vi "SFC_Rep Maintenance.vi"(5 "tblName":string, 6 "OperatorName":string, 7 "ModuleName":string, 8 "error in (no error)":errorcluster caption="错误输入（无错误）", 9 "Type":string, 10 ".NET:System.Data.DataSet":T1={"CaseSensitive"=FALSE, "Container"=refnum, "DataSetName"="", "DefaultViewManager"=refnum, "DesignMode"=FALSE, "EnforceConstraints"=FALSE, "ExtendedProperties"=refnum, "HasErrors"=FALSE, "IsInitialized"=FALSE, "Locale"=refnum, "Namespace"="", "Prefix"="", "Relations"=refnum, "RemotingFormat"=0, "SchemaSerializationMode"=1, "Site"=refnum, "Tables"=refnum} {"SchemaSerializationMode" items=["IncludeSchema"=1, "ExcludeSchema"=2]; "RemotingFormat" items=["Xml", "Binary"]}, 11 "Traceability 引用句柄":refnum<k24>) -> (0 "error out":errorcluster caption="错误输出", 2 ".NET:System.Data.DataSet":T1={"CaseSensitive"=FALSE, "Container"=refnum, "DataSetName"="", "DefaultViewManager"=refnum, "DesignMode"=FALSE, "EnforceConstraints"=FALSE, "ExtendedProperties"=refnum, "HasErrors"=FALSE, "IsInitialized"=FALSE, "Locale"=refnum, "Namespace"="", "Prefix"="", "Relations"=refnum, "RemotingFormat"=0, "SchemaSerializationMode"=1, "Site"=refnum, "Tables"=refnum} {"SchemaSerializationMode" items=["IncludeSchema"=1, "ExcludeSchema"=2]; "RemotingFormat" items=["Xml", "Binary"]}, 3 "Traceability 引用句柄输出":refnum<k24>)   [LabVIEW 2014, in "Traceability.lvlib"]
uses:
  Traceability.lvlib
  Traceability.dll
  System.Data
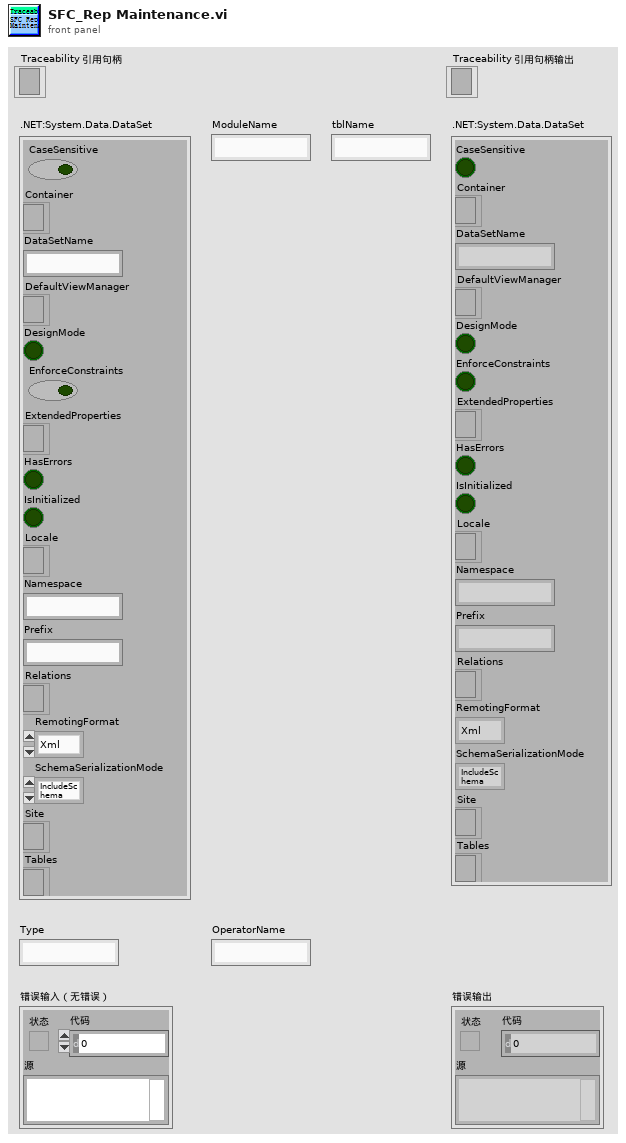
[diagram p1: front panel]
types:
  T1 = cluster{"CaseSensitive":bool, "Container":refnum<k24>, "DataSetName":string, "DefaultViewManager":refnum<k24>, "DesignMode":bool, "EnforceConstraints":bool, "ExtendedProperties":refnum<k24>, "HasErrors":bool, "IsInitialized":bool, "Locale":refnum<k24>, "Namespace":string, "Prefix":string, "Relations":refnum<k24>, "RemotingFormat":i32, "SchemaSerializationMode":i32, "Site":refnum<k24>, "Tables":refnum<k24>}
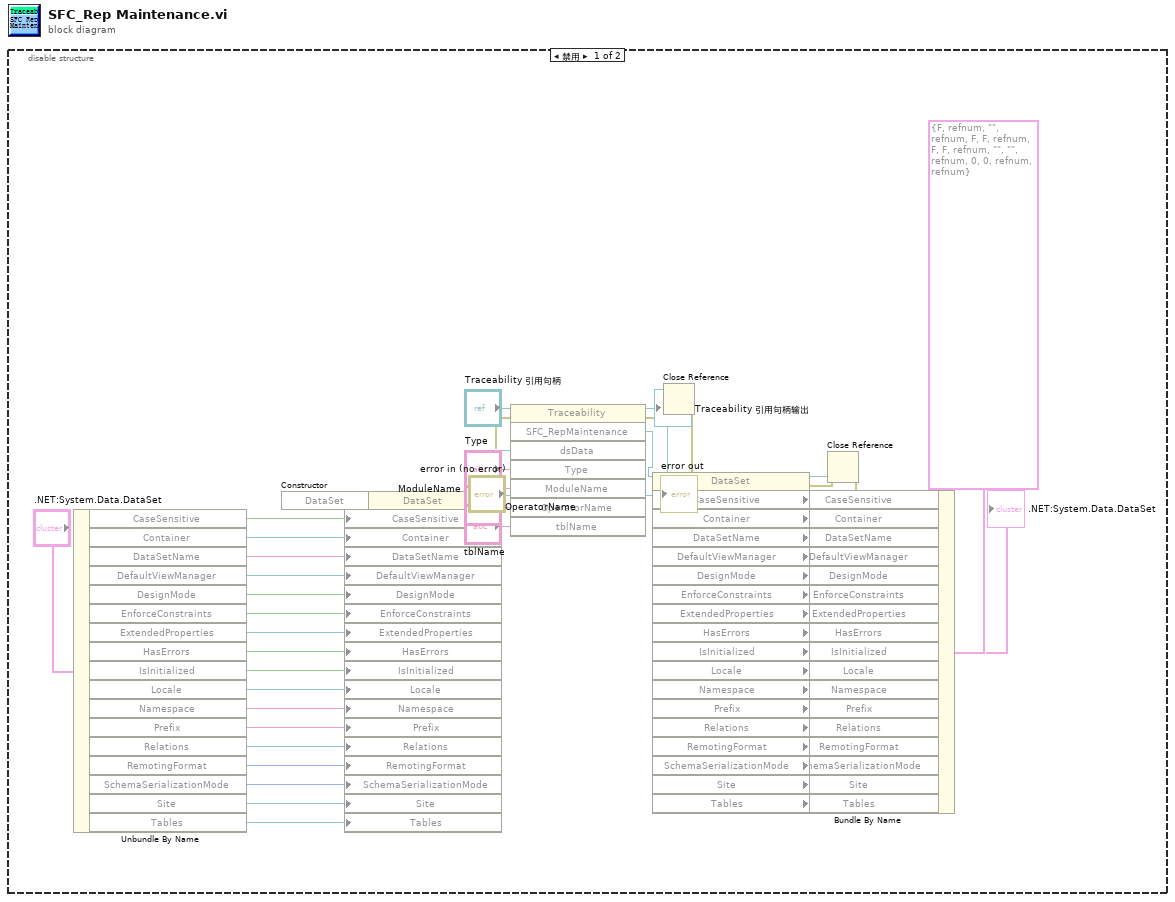
[diagram p0: block diagram]
diagram:
  n1 = disable-structure shown="禁用" {
    frame Disabled {
      n2 = Unbundle By Name(".NET:System.Data.DataSet") -> ("CaseSensitive"=w28:bool, "Container"=w27:refnum<k24>, "DataSetName"=w26:string, "DefaultViewManager"=w25:refnum<k24>, "DesignMode"=w24:bool, "EnforceConstraints"=w23:bool, "ExtendedProperties"=w22:refnum<k24>, "HasErrors"=w21:bool, "IsInitialized"=w20:bool, "Locale"=w19:refnum<k24>, "Namespace"=w18:string, "Prefix"=w17:string, "Relations"=w16:refnum<k24>, "RemotingFormat"=w15:i32, "SchemaSerializationMode"=w14:i32, "Site"=w13:refnum<k24>, "Tables"=w12:refnum<k24>)
      n3 = constructor class="DataSet"(error in="error in (no error)") -> (reference out=w32:refnum<k24>, error out=w31:errorcluster)  [unwired: 2 in, 1 out]
      n4 = property class="DataSet"(reference=w32, error in=w31, "CaseSensitive"=w28, "Container"=w27, "DataSetName"=w26, "DefaultViewManager"=w25, "DesignMode"=w24, "EnforceConstraints"=w23, "ExtendedProperties"=w22, "HasErrors"=w21, "IsInitialized"=w20, "Locale"=w19, "Namespace"=w18, "Prefix"=w17, "Relations"=w16, "RemotingFormat"=w15, "SchemaSerializationMode"=w14, "Site"=w13, "Tables"=w12) -> (reference out=w30:refnum<k24>, error out=w6:errorcluster)
      n5 = invoke class="Traceability" method="SFC_RepMaintenance"(reference="Traceability 引用句柄", error in=w6, "dsData"=w30, "Type"="Type", "ModuleName"="ModuleName", "OperatorName"="OperatorName", "tblName"="tblName") -> (reference out=→"Traceability 引用句柄输出":refnum<k24>, error out=w5:errorcluster, "SFC_RepMaintenance"=w52:refnum<k24>)  [unwired: 1 in, 5 out]
      n6 = Close Reference(reference=w30, error in (no error)=w5) -> (error out=w4:errorcluster)
      n7 = property class="DataSet"(reference=w52, error in=w4) -> (reference out=w3:refnum<k24>, error out=w2:errorcluster, "CaseSensitive"=w49:bool, "Container"=w48:refnum<k24>, "DataSetName"=w47:string, "DefaultViewManager"=w46:refnum<k24>, "DesignMode"=w45:bool, "EnforceConstraints"=w44:bool, "ExtendedProperties"=w43:refnum<k24>, "HasErrors"=w42:bool, "IsInitialized"=w41:bool, "Locale"=w40:refnum<k24>, "Namespace"=w39:string, "Prefix"=w38:string, "Relations"=w37:refnum<k24>, "RemotingFormat"=w36:i32, "SchemaSerializationMode"=w35:i32, "Site"=w34:refnum<k24>, "Tables"=w33:refnum<k24>)
      n8 = Bundle By Name(cluster=T1 {"CaseSensitive"=FALSE, "Container"=refnum, "DataSetName"="", "DefaultViewManager"=refnum, "DesignMode"=FALSE, "EnforceConstraints"=FALSE, "ExtendedProperties"=refnum, "HasErrors"=FALSE, "IsInitialized"=FALSE, "Locale"=refnum, "Namespace"="", "Prefix"="", "Relations"=refnum, "RemotingFormat"=0, "SchemaSerializationMode"=0, "Site"=refnum, "Tables"=refnum} (".NET:System.Data.DataSet"), "CaseSensitive"=w49, "Container"=w48, "DataSetName"=w47, "DefaultViewManager"=w46, "DesignMode"=w45, "EnforceConstraints"=w44, "ExtendedProperties"=w43, "HasErrors"=w42, "IsInitialized"=w41, "Locale"=w40, "Namespace"=w39, "Prefix"=w38, "Relations"=w37, "RemotingFormat"=w36, "SchemaSerializationMode"=w35, "Site"=w34, "Tables"=w33) -> (→".NET:System.Data.DataSet":T1)
      n9 = Close Reference(reference=w3, error in (no error)=w2) -> (error out=→"error out":errorcluster)
    }
    frame Enabled {
    }
  }
